vi "BuildCall.vi"(7 "PythonConverter_BD in":refnum<class "PyConvBD.lvclass">, 8 "error in":errorcluster, 11 "WhileLoop in":refnum<class "WhileLoop.lvclass">) -> (0 "error out":errorcluster, 3 "WhileLoop out":refnum<class "WhileLoop.lvclass">, 5 "PythonConverter_BD out":refnum<class "PyConvBD.lvclass">)   [LabVIEW 2014, in "Raspberry Pi Compatible Compiler for LabVIEW.lvlib" / "WhileLoop.lvclass"]
uses:
  WhileLoop.lvclass
  Python/PythonConverter_BD/PyConvBD.lvclass
  Python/Parsing/ListTypesTD.ctl
  Python/PythonConverter_BD/TypeDefs/NodeCall_TD.ctl
  Loop/Loop.lvclass/Loop.ctl
  ShiftRegister/ShiftRegister.lvclass/ShiftRegister.ctl
  RightShiftRegister/RightShiftRegister.lvclass
  LeftShiftRegister/LeftShiftRegister.lvclass
  LoopTunnel/LoopTunnel.lvclass
  Python/Parsing/Python Functions.lvlib
  Loop/Loop.lvclass
  ShiftRegister/ShiftRegister.lvclass
  Raspberry Pi Compatible Compiler for LabVIEW.lvlib
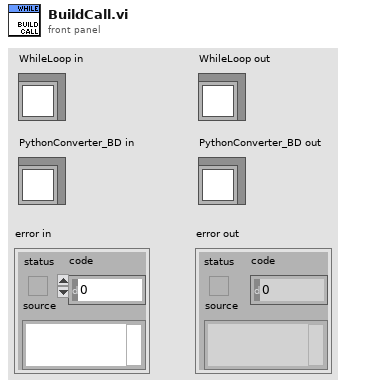
[diagram p1: front panel]
types:
  T1 = typedef "Raspberry Pi Compatible Compiler for LabVIEW.lvlib/NodeCall_TD.ctl" = cluster{"call":string, "collect":string, "Threaded":bool, "branches":string[]}
  T2 = typedef "Raspberry Pi Compatible Compiler for LabVIEW.lvlib/Python Functions.lvlib/ListTypesTD.ctl" = enum16{"list", "tuple", "parameter list", "output list", "return values"}
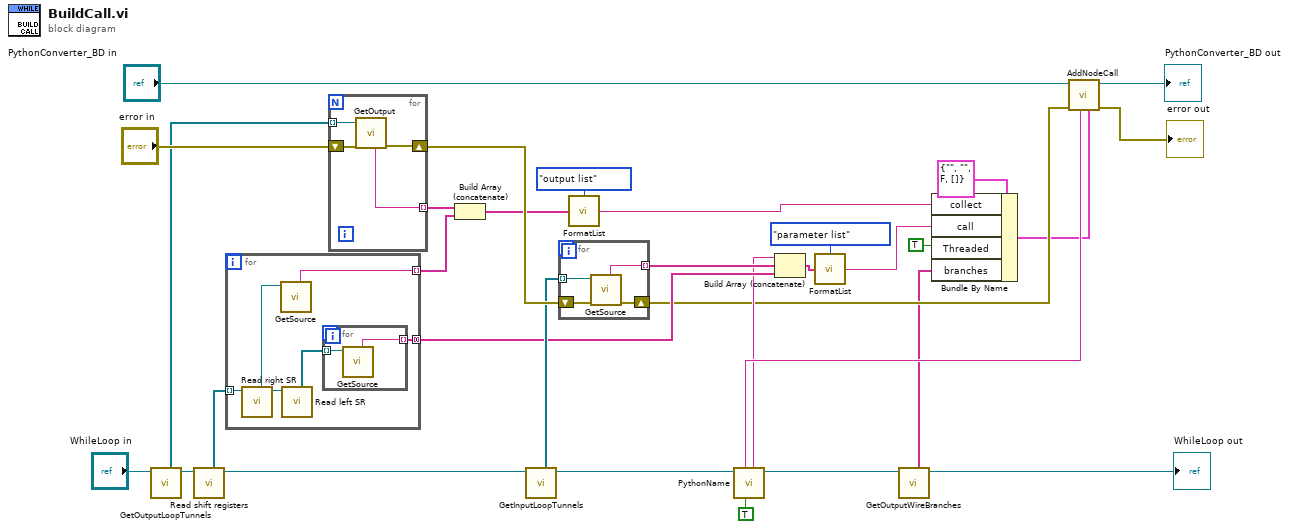
[diagram p0: block diagram]
diagram:
  n1 = call-dynamic "GetOutputLoopTunnels.vi"("Loop in"="WhileLoop in") -> ("Loop out"=w17:refnum<class "WhileLoop.lvclass">, "tunnels"=w19:refnum<class "LoopTunnel.lvclass">[])  [unwired: 6 in, 1 out]
  n2 = call "Read shift registers.vi"("Loop in"=w17) -> ("Loop out"=w16:refnum<class "WhileLoop.lvclass">, "shift registers"=w15:refnum<class "ShiftRegister.lvclass">[])  [unwired: 7 in]
  n3 = for {
    tunnel: w15 -> [w38] mode=indexing
    tunnel: [w36] -> w13 mode=indexing
    tunnel: [w33] -> w12 mode=concatenating
    n4 = call "Read right SR.vi"("ShiftRegister in"=w38) -> ("ShiftRegister out"=w35:refnum<class "ShiftRegister.lvclass">, "right SR"=w37:refnum<class "RightShiftRegister.lvclass">)  [unwired: 7 in]
    n5 = call-dynamic "GetSource.vi"("RightShiftRegister in"=w37) -> ("name"=w36:string)  [unwired: 6 in, 2 out]
    n6 = call "Read left SR.vi"("ShiftRegister in"=w35) -> ("left SR"=w34:refnum<class "LeftShiftRegister.lvclass">[])  [unwired: 7 in, 1 out]
    n7 = for {
      tunnel: w34 -> [w40] mode=indexing
      tunnel: [w39] -> w33 mode=indexing
      n8 = call-dynamic "GetSource.vi"("LeftShiftRegister in"=w40) -> ("name"=w39:string)  [unwired: 6 in, 2 out]
    }
  }
  n9 = for {
    tunnel: w19 -> [w44] mode=indexing
    shift-right: [w41] -> w28
    shift-left: "error in" -> [w43]
    tunnel: [w42] -> w32 mode=indexing
    n10 = call-dynamic "GetOutput.vi"("error in"=w43, "Tunnel in"=w44) -> ("error out"=w41:errorcluster, "name"=w42:string)  [unwired: 5 in, 1 out]
  }
  n11 = Build Array (concatenate)(w32, w13) -> (w14:string[])
  n12 = call-dynamic "GetInputLoopTunnels.vi"("Loop in"=w16) -> ("Loop out"=w11:refnum<class "WhileLoop.lvclass">, "tunnels"=w18:refnum<class "LoopTunnel.lvclass">[])  [unwired: 6 in, 1 out]
  n13 = for {
    tunnel: w18 -> [w48] mode=indexing
    shift-right: [w46] -> w9
    shift-left: w28 -> [w47]
    tunnel: [w45] -> w22 mode=indexing
    n14 = call-dynamic "GetSource.vi"("error in"=w47, "Tunnel in"=w48) -> ("error out"=w46:errorcluster, "name"=w45:string)  [unwired: 5 in, 1 out]
  }
  n15 = call "FormatList.vi"("values"=w14, "type"=ListTypesTD."output list") -> ("python object"=w6:string)
  n16 = call-dynamic "PythonName.vi"("add self"=TRUE, "Node in"=w11) -> ("Node out"=w3:refnum<class "WhileLoop.lvclass">, "name"=w10:string, "UID"=w29:string)  [unwired: 6 in, 1 out]
  n17 = Build Array (concatenate)(w10, w22, w12) -> (w21:string[])
  n18 = call "FormatList.vi"("values"=w21, "type"=ListTypesTD."parameter list") -> ("python object"=w5:string)
  n19 = call-dynamic "GetOutputWireBranches.vi"("Loop in"=w3) -> ("Loop out"=→"WhileLoop out":refnum<class "WhileLoop.lvclass">, "branches"=w1:string[])  [unwired: 6 in, 1 out]
  n20 = Bundle By Name(cluster=T1 {"call"="", "collect"="", "Threaded"=FALSE, "branches"=[]} ("call"), "collect"=w6, "call"=w5, "Threaded"=TRUE, "branches"=w1) -> (w4:T1)
  n21 = call "AddNodeCall.vi"("call"=w4, "name"=w29, "error in"=w9, "PythonConverter_BD in"="PythonConverter_BD in") -> ("error out"=→"error out":errorcluster, "PythonConverter_BD out"=→"PythonConverter_BD out":refnum<class "PyConvBD.lvclass">)  [unwired: 4 in]
